vi "Frequency Domain Calibration.vi"(0 "spectra in":T2(array[cluster]), 1 "ranges to calibrate [%]":dbl[](array[numeric]), 2 "frequencies to calibrate [Hz]":dbl[](array[numeric]), 5 "gains":dbl[][][](array[numeric]), 7 "phase delays [deg]":dbl[][][](array[numeric]), 9 "system info in":refnum<class "EP System Info.lvclass">, 11 "error in (no error)":errorcluster, 12 "actual ranges [%]":dbl[](array[numeric])) -> (4 "spectra out":T2(array[cluster]), 10 "system info out":refnum<class "EP System Info.lvclass">, 15 "error out":errorcluster)   [LabVIEW 2014, in "NI_EP_Power Quality.lvlib"]
doc: "Calibrates a phase spectrum by applying gains and phase delays at all frequency bins, based on <B>actual ranges</B>. You can use the Get Range Utilization VI to calculate range utilization. You must specify <B>frequencies to calibrate</B> and <B>ranges to calibrate</B> in ascending order.\n\nThis VI supports measuring single-line and multiple-line systems."
uses:
  <vilib>/addons/Electrical Power/PQ/NI_EP_Power Quality.lvlib
  <vilib>/addons/Electrical Power/PQ/Common/Controls/ep_AI Data Channel.ctl
  <vilib>/addons/Electrical Power/PQ/Common/Classes/System Info/EP System Info.lvclass
  <vilib>/addons/Electrical Power/PQ/Scaling_Calibration/subVIs/ep_Compute Third Current (Spectra).vi
  <vilib>/Analysis/NI_AALPro.lvlib
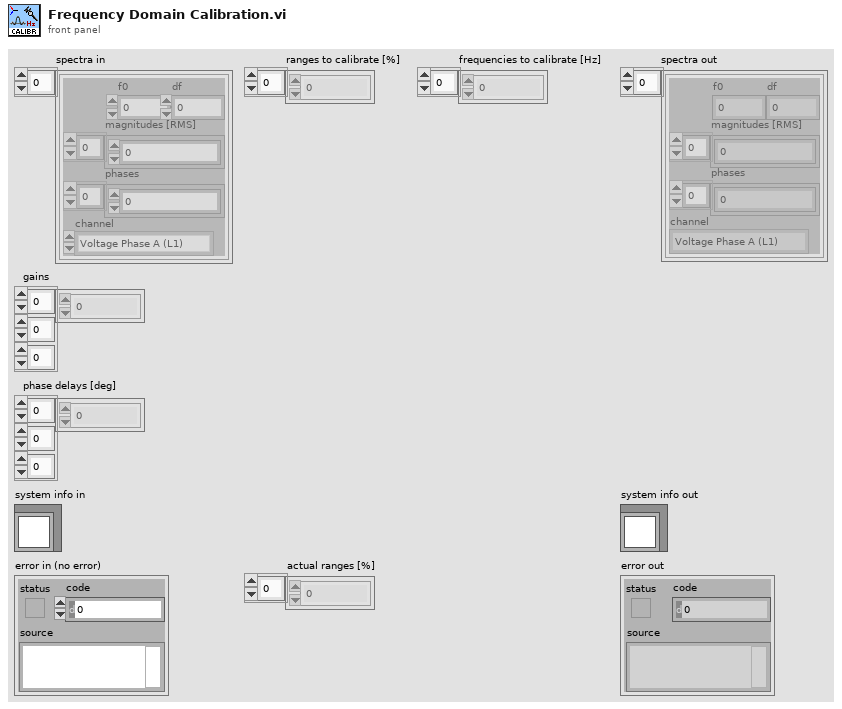
[diagram p1: front panel]
types:
  T1 = typedef "NI_EP_Power Quality.lvlib/ep_AI Data Channel.ctl" = enum16{"Voltage Phase A (L1)", "Voltage Phase B (L2)", "Voltage Phase C (L3)", "Voltage Phase N (Neutral)", "Current Phase A (L1)", "Current Phase B (L2)", "Current Phase C (L3)", "Current Phase N (Neutral)"}
  T2 = cluster{"f0":dbl, "df":dbl, "magnitudes [RMS]":dbl[], "phases":dbl[], "channel":T1}[]
  T3 = cluster{"f0":dbl, "df":dbl, "magnitudes [RMS]":dbl[], "phases":dbl[], "channel":T1}
  T4 = typedef "NI_EP_Power Quality.lvlib/ep_Wiring.ctl" = enum16{"4xUph + 4xI", "3xUph + 4xI", "3xUline + 4xI", "3xUph + 3xI", "3xUline + 3xI", "3xUph + 2xI", "3xUline + 2xI", "1xUph + 1xI"}
  T5 = cluster{"f0":dbl, "df":dbl, "magnitude":dbl[], "phase":dbl[], "channel":T1}[]
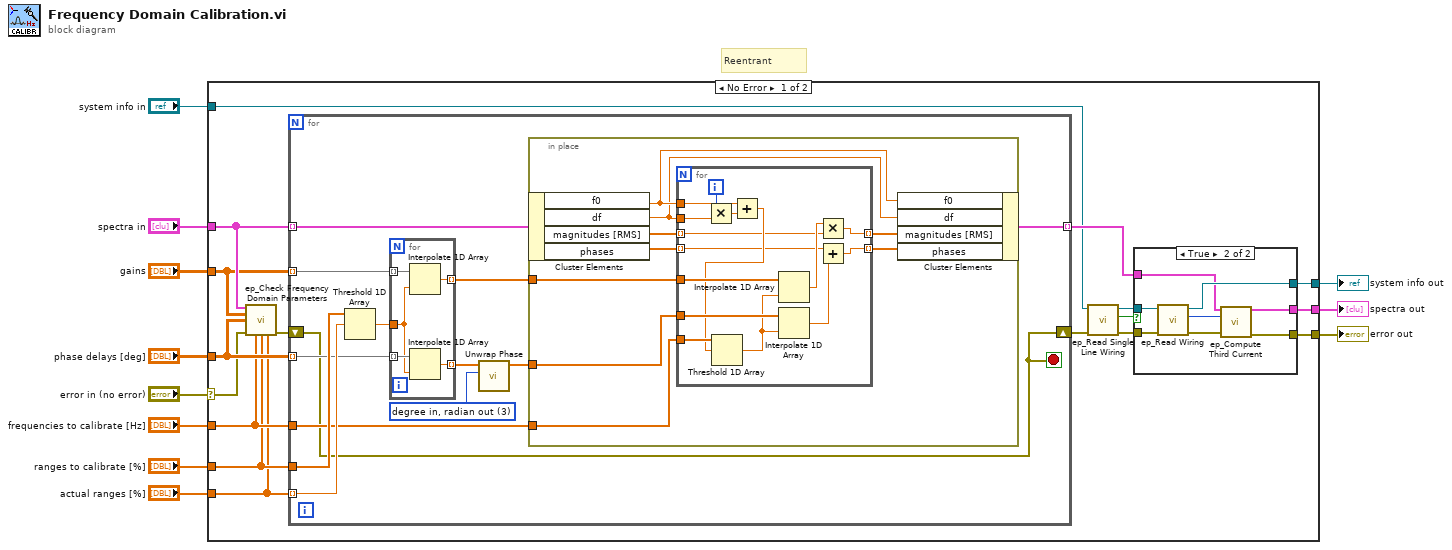
[diagram p0: block diagram]
diagram:
  # "Reentrant"
  n1 = case shown="No Error" "error in (no error)" {
    selector: "error in (no error)" -> [w13 w82]
    tunnel: [w28 w83] -> w11
    tunnel: [w27 w82] -> w10
    tunnel: [w26 w84] -> w9
    tunnel: "spectra in" -> [w25 w83]
    tunnel: "gains" -> [w24 _]
    tunnel: "phase delays [deg]" -> [w23 _]
    tunnel: "frequencies to calibrate [Hz]" -> [w22 _]
    tunnel: "ranges to calibrate [%]" -> [w21 _]
    tunnel: "actual ranges [%]" -> [w20 _]
    tunnel: "system info in" -> [w12 w84]
    frame No Error {
      n2 = call <vilib>:"ep_Check Frequency Domain Parameters.vi"("spectra in"=w25, "gains"=w24, "phase delays [deg]"=w23, "error in (no error)"=w13, "frequencies to calibrate [Hz]"=w22, "ranges to calibrate [%]"=w21, "actual ranges [%]"=w20) -> ("error out"=w19:errorcluster)  [unwired: 8 in]
      n3 = for {
        tunnel: w20 -> [w51] mode=indexing
        tunnel: w21 -> [w52]
        tunnel: w25 -> [w50] mode=indexing
        tunnel: w23 -> [w43] mode=indexing
        tunnel: w22 -> [w48]
        tunnel: [w47] -> w15 mode=indexing
        tunnel: w24 -> [w42] mode=indexing
        shift-right: [w40] -> w16
        shift-left: w19 -> [w40]
        stop <- w40 stop-if-true
        w44 = 3 items=["radian in, radian out", "radian in, degree out", "degree in, degree out", "degree in, radian out"] ("phase unit")
        n4 = Threshold 1D Array(2:w51, 3:w52) -> (0:w49:dbl)  [unwired: 1 in]
        n5 = for {
          tunnel: w43 -> [w57] mode=indexing
          tunnel: w49 -> [w53]
          tunnel: [w56] -> w45 mode=indexing
          tunnel: w42 -> [w54] mode=indexing
          tunnel: [w55] -> w41 mode=indexing
          n6 = Interpolate 1D Array(1:w53, 2:w54) -> (0:w55:dbl)
          n7 = Interpolate 1D Array(1:w53, 2:w57) -> (0:w56:dbl)
        }
        n8 = call <vilib>:"Unwrap Phase.vi"("phase unit"=w44, "Phase"=w45) -> ("Unwrapped Phase"=w46:dbl[])  [unwired: 8 in, 1 out]
        n9 = in-place {
          in-place-border: w46 -> [w64]
          in-place-border: w48 -> [w63]
          in-place-border: w41 -> [w62]
          n10 = in-place-cluster #1(w50) -> ("f0"=w66:dbl, "df"=w65:dbl, "magnitudes [RMS]"=w61:dbl[], "phases"=w60:dbl[])
          n11 = for {
            tunnel: w61 -> [w70] mode=indexing
            tunnel: w66 -> [w79]
            tunnel: w65 -> [w78]
            tunnel: w64 -> [w76]
            tunnel: w63 -> [w77]
            tunnel: w62 -> [w74]
            tunnel: w60 -> [w69] mode=indexing
            tunnel: [w68] -> w59 mode=indexing
            tunnel: [w67] -> w58 mode=indexing
            i -> [w81]
            n12 = Multiply(x=w81, y=w78) -> (x*y=w80:dbl)
            n13 = Add(x=w79, y=w80) -> (x+y=w71:dbl)
            n14 = Threshold 1D Array(2:w71, 3:w77) -> (0:w73:dbl)  [unwired: 1 in]
            n15 = Interpolate 1D Array(1:w73, 2:w74) -> (0:w72:dbl)
            n16 = Interpolate 1D Array(1:w73, 2:w76) -> (0:w75:dbl)
            n17 = Multiply(x=w72, y=w70) -> (x*y=w68:dbl)
            n18 = Add(x=w69, y=w75) -> (x+y=w67:dbl)
          }
          n19 = in-place-cluster #1("f0"=w66, "df"=w65, "magnitudes [RMS]"=w59, "phases"=w58) -> (w47:T3)
        }
      }
      n20 = call <vilib>:"ep_Read Single Line Wiring.vi"("error in (no error)"=w16, "system info in"=w12) -> ("error out"=w17:errorcluster, "single line wiring? (F)"=w14:bool, "system info out"=w18:refnum<class "EP System Info.lvclass">)  [unwired: 7 in]
      n21 = case shown="True" w14 {
        tunnel: [w30 w39] -> w28
        tunnel: [w29 w38] -> w27
        tunnel: [w31 w37] -> w26
        tunnel: w18 -> [w31 w34]
        tunnel: w17 -> [w29 w33]
        tunnel: w15 -> [w30 w32]
        frame False {
        }
        frame True {
          n22 = call <vilib>:"ep_Read Wiring.vi"("error in (no error)"=w33, "system info in"=w34) -> ("error out"=w35:errorcluster, "wiring"=w36:T4, "system info out"=w37:refnum<class "EP System Info.lvclass">)  [unwired: 6 in, 1 out]
          n23 = call-poly <vilib>:"ep_Compute Third Current.vi"("complex current spectra in (5Hz step)"=w32, "wiring"=w36, "error in (no error)"=w35) -> ("complex current spectra out (5Hz step)"=w39:T5, "error out"=w38:errorcluster)  [unwired: 11 in]
        }
      }
    }
    frame Error {
    }
  }
  "error out" <- w10
  "spectra out" <- w11
  "system info out" <- w9
